vi "AAL LP Kaiser Window Design.vi"(8 "A stop [dB]":dbl=72.0 format="%.2f", 9 "stopband":dbl=0.25 format="%.2f", 10 "passband":dbl=0.05 format="%.2f", 11 "fs":dbl=1.0 format="%.2f") -> (0 "error":i32, 2 "taps":i32, 3 "filter coefficients":dbl[](array[numeric]) format="%.2f")   [LabVIEW 2020, in "NI_AALPro.lvlib"]
uses:
  <vilib>/Analysis/NI_AALPro.lvlib
  <vilib>/Analysis/4window.llb/Kaiser-Bessel Window (DBL).vi
  <vilib>/Analysis/NI_AALBase.lvlib
panel:
  out "Waveform Graph":T1(graph)
  in  "debug?":bool
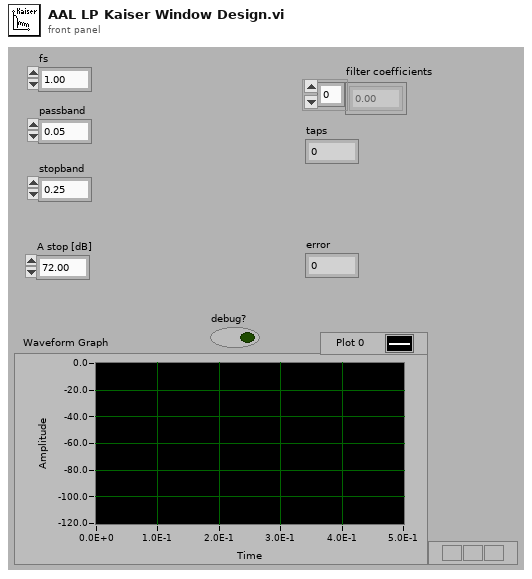
[diagram p1: front panel]
types:
  T1 = cluster{"Lower Freq":dbl, "df":dbl, "amplitude":dbl[]}
  T2 = enum32{"None", "Hanning", "Hamming", "Triangular", "Blackman", "Exact Blackman", "Blackman-Harris", "Kaiser-Bessel", "Flat Top"}
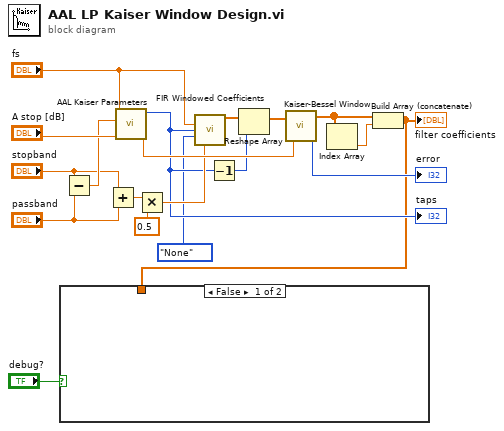
[diagram p0: block diagram]
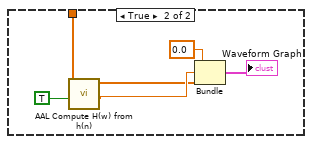
[diagram p2: hidden frame]
diagram:
  n1 = Subtract(x="stopband", y="passband") -> (x-y=w14:dbl)
  n2 = Add(x="stopband", y="passband") -> (x+y=w8:dbl)
  n3 = call <vilib>:"AAL Kaiser Parameters.vi"("A stop [dB]"="A stop [dB]", "delta f"=w14, "fs"="fs") -> ("beta"=w15:dbl, "taps"=w5:i32)  [unwired: 7 in]
  "taps" <- w5
  n4 = Multiply(x=w8, y=0.5) -> (x*y=w10:dbl)
  n5 = call <vilib>:"FIR Windowed Coefficients.vi"("sampling freq: fs"="fs", "taps"=w5, "window"=T2."None", "low cutoff freq: fl"=w10) -> ("FIR Windowed Coefficients"=w7:dbl[])  [unwired: 10 in, 1 out]
  n6 = Decrement(x=w5) -> (x-1=w4:i32)
  n7 = Reshape Array(w7, w4) -> (w6:dbl[])
  n8 = call-poly <vilib>:"Kaiser-Bessel Window.vi"("beta"=w15, "X"=w6) -> ("error"=→"error":i32, "Windowed X"=w18:dbl[])
  n9 = Index Array(array=w18) -> (element=w17:dbl)  [unwired: 1 in]
  n10 = Build Array (concatenate)(w18, w17) -> (w1:dbl[])
  "filter coefficients" <- w1
  n11 = case shown="False" "debug?" {
    tunnel: w1 -> [_ w20]
    frame False {
    }
    frame True {
      n12 = call <vilib>:"AAL Compute H(w) from h(n).vi"("dB on?"=TRUE, "h[n]"=w20) -> ("df"=w24:dbl, "amplitude"=w21:dbl[])  [unwired: 7 in, 1 out]
      n13 = Bundle("Lower Freq"=0.0, "df"=w24, "amplitude"=w21) -> (→"Waveform Graph":T1)  [unwired: 1 in]
    }
  }
